vi "Open Client Connection.vi"(8 "error in (no error)":errorcluster, 9 "Port":u16, 10 "address":string, 11 "RemoteControl.ZMQ in":refnum<class "RemoteControl.ZMQ.lvclass">) -> (0 "error out":errorcluster, 3 "RemoteControl.ZMQ out":refnum<class "RemoteControl.ZMQ.lvclass">)   [LabVIEW 2019, in "RemoteControl.ZMQ.lvclass"]
uses:
  RemoteControl.ZMQ.lvclass
  RemoteControl.ZMQ.lvclass/RemoteControl.ZMQ.ctl
  <vilib>/addons/zeromq/socket_type.ctl
  RemoteControl/RemoteControl.lvclass
  <vilib>/addons/zeromq/zmq_context.lvclass
  <vilib>/addons/zeromq/zeromq.lvlib
  <vilib>/addons/zeromq/zmq_socket.lvclass
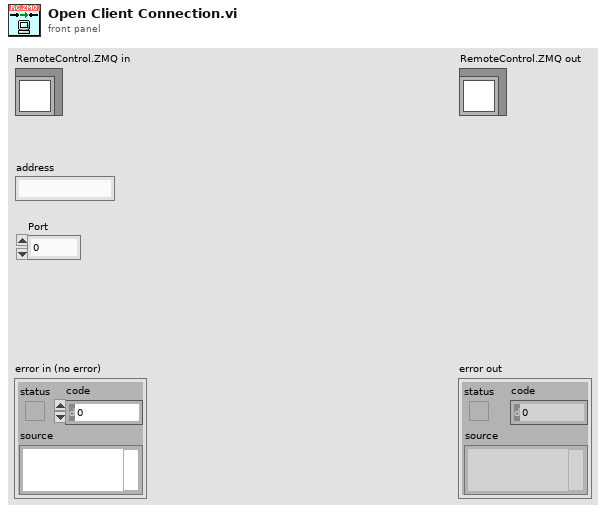
[diagram p1: front panel]
types:
  T1 = typedef "zeromq.lvlib/socket_type.ctl" = enum8{"ZMQ_PAIR", "ZMQ_PUB", "ZMQ_SUB", "ZMQ_REQ", "ZMQ_REP", "ZMQ_DEALER", "ZMQ_ROUTER", "ZMQ_PULL", "ZMQ_PUSH", "ZMQ_XPUB", "ZMQ_XSUB", "ZMQ_STREAM", "ZMQ_SERVER", "ZMQ_CLIENT", "ZMQ_RADIO", "ZMQ_DISH", "ZMQ_GATHER", "ZMQ_SCATTER", "ZMQ_DGRAM"}
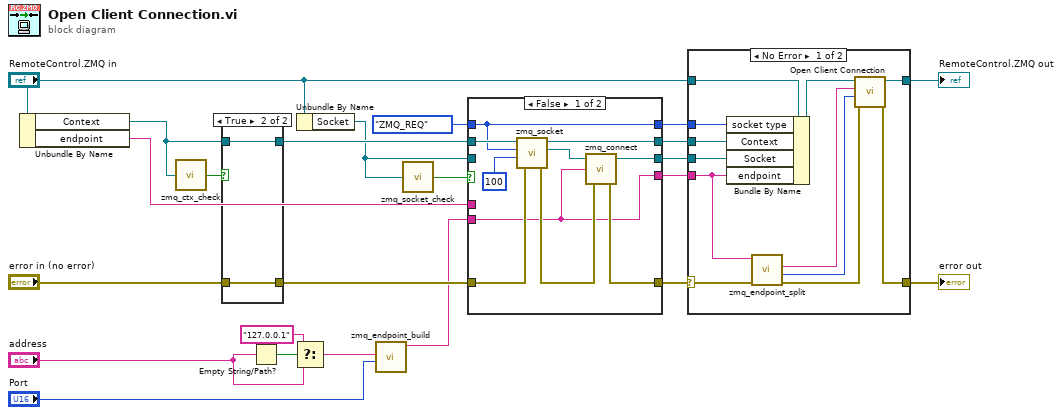
[diagram p0: block diagram]
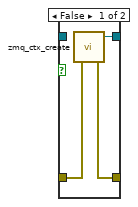
[diagram p3: hidden frame]
diagram:
  n1 = Unbundle By Name("RemoteControl.ZMQ in") -> ("Context"=w11:refnum<class "zmq_context.lvclass">, "endpoint"=w1:string)
  n2 = call <vilib>:"zmq_ctx_check.vi"("context in"=w11) -> ("valid?"=w18:bool)
  n3 = case shown="True" w18 {
    tunnel: "error in (no error)" -> [w26 w27]
    tunnel: [w25 w28] -> w20
    tunnel: [w24 w27] -> w17
    tunnel: w11 -> [_ w28]
    frame False {
      n4 = call <vilib>:"zmq_ctx_create.vi"("error in"=w26) -> ("error out"=w24:errorcluster, "context out"=w25:refnum<class "zmq_context.lvclass">)  [unwired: 3 in]
    }
    frame True {
    }
  }
  n5 = Empty String/Path?(string/path="address") -> (empty?=w10:bool)
  n6 = Select(t="127.0.0.1", s=w10, f="address") -> (s? t:f=w7:string)
  n7 = Unbundle By Name("RemoteControl.ZMQ in") -> ("Socket"=w12:refnum<class "zmq_socket.lvclass">)
  n8 = call <vilib>:"zmq_endpoint_build.vi"("port"="Port", "address"=w7) -> ("endpoint"=w3:string)  [unwired: 3 in, 2 out]
  n9 = call <vilib>:"zmq_socket_check.vi"("socket in"=w12) -> ("valid?"=w15:bool)
  n10 = case shown="False" w15 {
    tunnel: w20 -> [w38 w43]
    tunnel: [w37 w43] -> w19
    tunnel: [w32 w41] -> w5
    tunnel: [w30 w40] -> w4
    tunnel: w17 -> [w36 w40]
    tunnel: socket_type."ZMQ_REQ" ("socket type") -> [w35 w42]
    tunnel: w12 -> [_ w41]
    tunnel: [w35 w42] -> w13
    tunnel: w3 -> [w29 _]
    tunnel: [w29 w39] -> w2
    tunnel: w1 -> [_ w39]
    frame False {
      n11 = call <vilib>:"zmq_socket.vi"("error in"=w36, "linger (ms)"=100, "socket type"=w35, "context in"=w38) -> ("error out"=w31:errorcluster, "socket out"=w33:refnum<class "zmq_socket.lvclass">, "context out"=w37:refnum<class "zmq_context.lvclass">)  [unwired: 1 in]
      n12 = call <vilib>:"zmq_connect.vi"("error in"=w31, "endpoint"=w29, "socket in"=w33) -> ("error out"=w30:errorcluster, "socket out"=w32:refnum<class "zmq_socket.lvclass">)  [unwired: 1 in]
    }
    frame True {
    }
  }
  n13 = case shown="No Error" w4 {
    selector: w4 -> [w45 w57]
    tunnel: w13 -> [w55 _]
    tunnel: w2 -> [w48 _]
    tunnel: w19 -> [w54 _]
    tunnel: [w52 w57] -> w22
    tunnel: "RemoteControl.ZMQ in" -> [w51 w56]
    tunnel: [w50 w56] -> w21
    tunnel: w5 -> [w49 _]
    frame No Error {
      n14 = Bundle By Name(cluster=w51, "socket type"=w55, "Context"=w54, "Socket"=w49, "endpoint"=w48) -> (w53:refnum<class "RemoteControl.ZMQ.lvclass">)
      n15 = call <vilib>:"zmq_endpoint_split.vi"("error in"=w45, "endpoint"=w48) -> ("error out"=w44:errorcluster, "port"=w47:u16, "address"=w46:string)  [unwired: 2 in, 1 out]
      n16 = call-parent "Open Client Connection.vi"("error in (no error)"=w44, "Port"=w47, "address"=w46, "RemoteControl in"=w53) -> ("error out"=w52:errorcluster, "RemoteControl out"=w50:refnum<class "RemoteControl.ZMQ.lvclass">)  [unwired: 6 in]
    }
    frame Error {
    }
  }
  "error out" <- w22
  "RemoteControl.ZMQ out" <- w21
